vi "Write selectedEdge.vi"(8 "error in (no error)":errorcluster, 10 "selectedEdge":i32, 11 "FSM.Graph in":refnum<class "FSM.Graph.lvclass">) -> (0 "error out":errorcluster, 3 "FSM.Graph out":refnum<class "FSM.Graph.lvclass">)   [LabVIEW 2020, in "FSM.Graph.lvclass"]
uses:
  FSM.Graph.lvclass
  FSM.Graph.lvclass/FSM.Graph.ctl
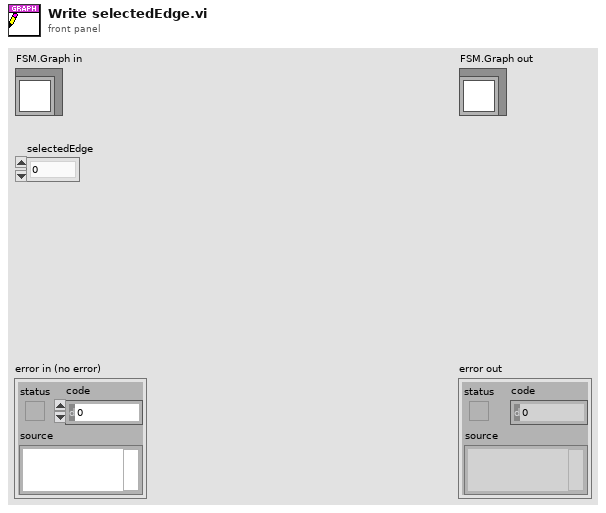
[diagram p1: front panel]
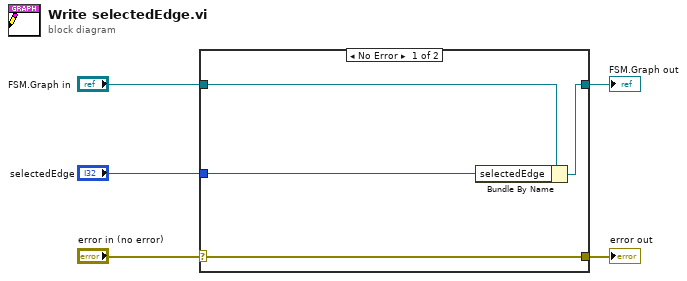
[diagram p0: block diagram]
diagram:
  n1 = case shown="No Error" "error in (no error)" {
    selector: "error in (no error)" -> [w9 w10]
    tunnel: [w9 w10] -> w4
    tunnel: [w7 w11] -> w2
    tunnel: "FSM.Graph in" -> [w8 w11]
    tunnel: "selectedEdge" -> [w6 _]
    frame No Error {
      n2 = Bundle By Name(cluster=w8, "selectedEdge"=w6) -> (w7:refnum<class "FSM.Graph.lvclass">)
    }
    frame Error {
    }
  }
  "error out" <- w4
  "FSM.Graph out" <- w2
